vi "EncoderSetting.vi"(1 "Line Count (Encoder)":dbl) -> (0 "DistancePerCount":dbl)   [LabVIEW 2015]
doc: "This VI will calculate DistancePerCount for an encoder on the Rhino tracks. (3in Wheel diameter)"
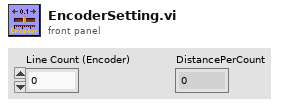
[diagram p1: front panel]
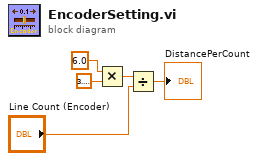
[diagram p0: block diagram]
diagram:
  n1 = Multiply(x=6.0, y=3.141592653589793) -> (x*y=w2:dbl)
  n2 = Divide(x=w2, y="Line Count (Encoder)") -> (x/y=→"DistancePerCount":dbl)
